vi "xml_to_dictionary.vi"(8 "error in (no error)":errorcluster, 11 "XML File Path":path) -> (0 "error out":errorcluster, 3 "units []":T1[](array[typedef]))   [LabVIEW 2015, in "lv-unit-conversion.lvlib"]
uses:
  lv-unit-conversion.lvlib
  public/_controls/unit.ctl
  public/_controls/error.ctl
  <vilib>/xml/Load XML File.vi
  <vilib>/xml/Close Reference(Node).vi
  <vilib>/xml/NI_XML.lvlib
  <resource>/objmgr/DOMUserDefRef.rc
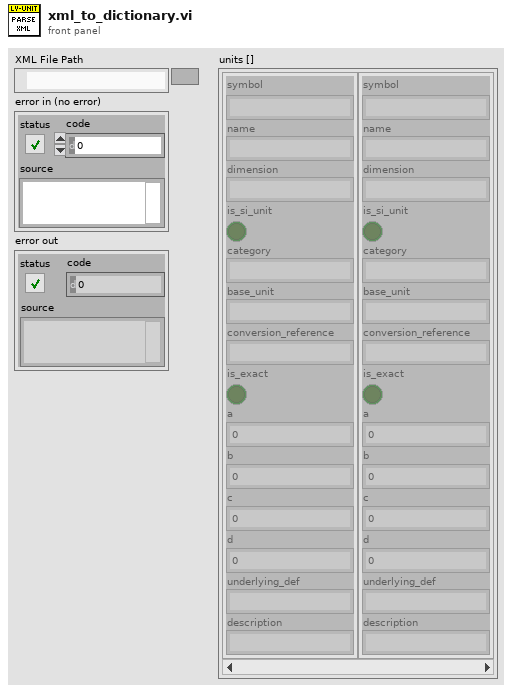
[diagram p1: front panel]
types:
  T1 = typedef "lv-unit-conversion.lvlib/unit.ctl" = cluster{"symbol":string, "name":string, "dimension":string, "is_si_unit":bool, "category":string, "base_unit":string, "conversion_reference":string, "is_exact":bool, "a":dbl, "b":dbl, "c":dbl, "d":dbl, "underlying_def":string, "description":string}
  T2 = typedef "lv-unit-conversion.lvlib/error.ctl" = enum16{"<lv-unit-conversion_error>", "unit_not_found", "xml_parser", "<null>"}
  T3 = cluster{cluster{"Name":string, "Value":string}[]}
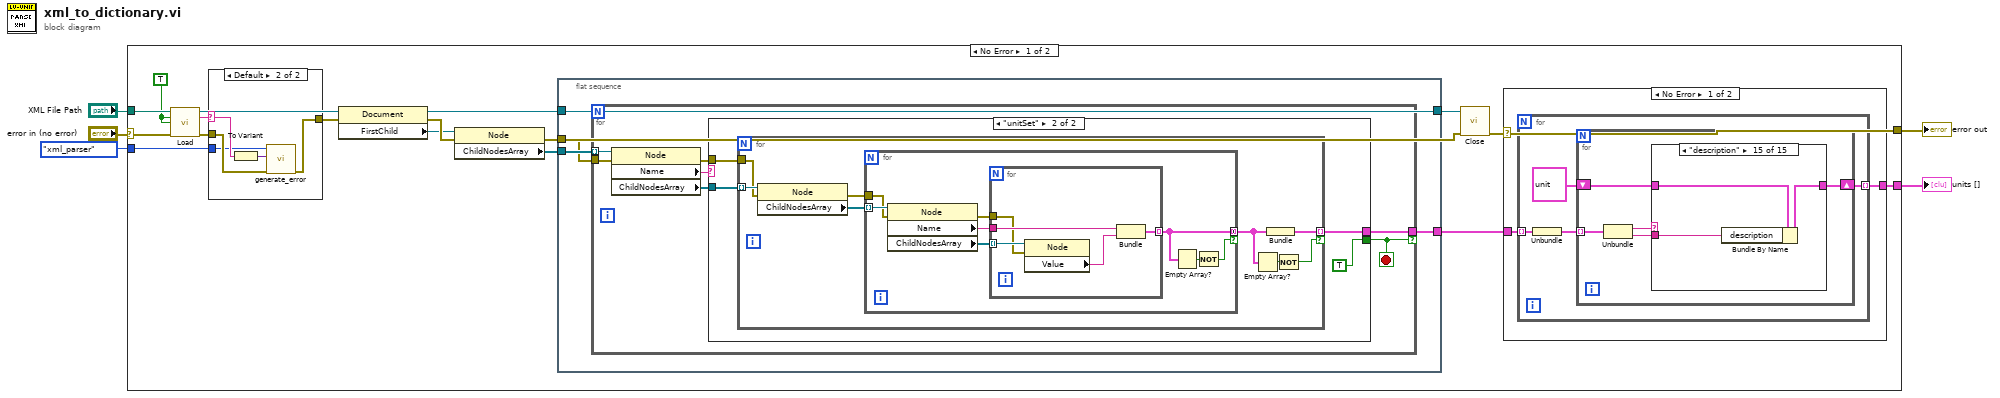
[diagram p0: block diagram]
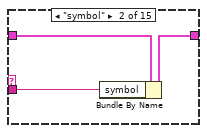
[diagram p3: hidden frame]
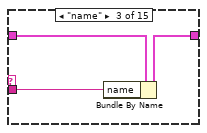
[diagram p4: hidden frame]
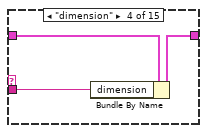
[diagram p5: hidden frame]
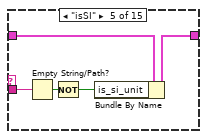
[diagram p6: hidden frame]
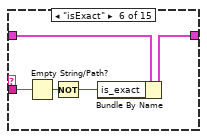
[diagram p7: hidden frame]
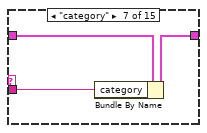
[diagram p8: hidden frame]
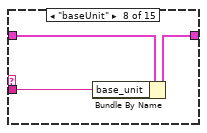
[diagram p9: hidden frame]
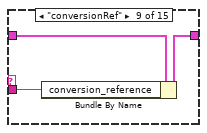
[diagram p10: hidden frame]
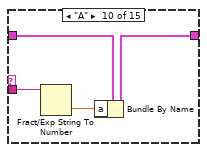
[diagram p11: hidden frame]
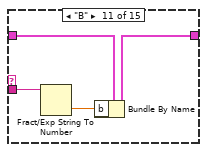
[diagram p12: hidden frame]
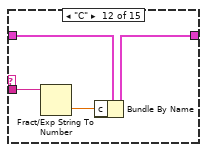
[diagram p13: hidden frame]
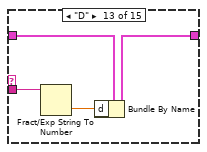
[diagram p14: hidden frame]
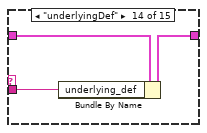
[diagram p15: hidden frame]
diagram:
  n1 = case shown="No Error" "error in (no error)" {
    selector: "error in (no error)" -> [w13 w127]
    tunnel: "XML File Path" -> [w22 _]
    tunnel: [w7 w127] -> w4
    tunnel: error."xml_parser" ("error") -> [w9 _]
    tunnel: [w6 _] -> w1
    frame No Error {
      w21 = TRUE ("process namespaces (False)")
      n2 = call-poly <vilib>:"Load.vi"("path to XML document"=w22, "process namespaces (False)"=w21, "process schema (False)"=w21, "error in (no error)"=w13) -> ("DOM document out"=w20:refnum<k20>, "parse errors"=w12:string, "error out"=w11:errorcluster)  [unwired: 9 in]
      n3 = case shown="Default" w12 {
        selector: w12 -> [_ w90]
        tunnel: w11 -> [w85 w89]
        tunnel: [w85 w88] -> w10
        tunnel: w9 -> [_ w87]
        frame "" {
        }
        frame Default {
          n4 = To Variant(anything=w90) -> (Variant=w86:variant)
          n5 = call "generate_error.vi"("error in (no error)"=w89, "data"=w86, "error"=w87) -> ("error out"=w88:errorcluster)  [unwired: 8 in]
        }
      }
      n6 = property class="Document"(reference=w20, error in=w10) -> (reference out=w16:refnum<k20>, error out=w18:errorcluster, "FirstChild"=w17:refnum<k20>)
      n7 = property class="Node"(reference=w17, error in=w18) -> (error out=w14:errorcluster, "ChildNodesArray"=w19:refnum<k20>[])  [unwired: 1 out]
      n8 = flat-sequence {
        tunnel: w19 -> [w94]
        tunnel: [w93] -> w8
        tunnel: w16 -> [w92]
        tunnel: [w92] -> w15
        tunnel: w14 -> [w91]
        frame #0 {
          n9 = for {
            tunnel: w94 -> [w101] mode=indexing
            tunnel: [w97] -> w93 if=w95
            tunnel: w91 -> [w100]
            stop <- w95 stop-if-true
            n10 = property class="Node"(reference=w101, error in=w100) -> (error out=w98:errorcluster, "Name"=w96:string, "ChildNodesArray"=w99:refnum<k20>[])  [unwired: 1 out]
            n11 = case shown="\"unitSet\"" w96 {
              tunnel: w99 -> [_ w105]
              tunnel: w98 -> [_ w104]
              tunnel: [_ w103] -> w97
              tunnel: [_ TRUE] -> w95
              frame "False", Default {
              }
              frame "unitSet" {
                n12 = for {
                  tunnel: w105 -> [w113] mode=indexing
                  tunnel: [w109] -> w103 mode=indexing if=w110
                  tunnel: w104 -> [w107]
                  n13 = property class="Node"(reference=w113, error in=w107) -> (error out=w106:errorcluster, "ChildNodesArray"=w112:refnum<k20>[])  [unwired: 1 out]
                  n14 = for {
                    tunnel: w112 -> [w121] mode=indexing
                    tunnel: [w117] -> w108 mode=concatenating if=w116
                    tunnel: w106 -> [w115]
                    n15 = property class="Node"(reference=w121, error in=w115) -> (error out=w114:errorcluster, "Name"=w119:string, "ChildNodesArray"=w120:refnum<k20>[])  [unwired: 1 out]
                    n16 = for {
                      tunnel: w120 -> [w126] mode=indexing
                      tunnel: w119 -> [w123]
                      tunnel: [w124] -> w117 mode=indexing
                      tunnel: w114 -> [w122]
                      n17 = property class="Node"(reference=w126, error in=w122) -> ("Value"=w125:string)  [unwired: 2 out]
                      n18 = Bundle("Name"=w123, "Value"=w125) -> (w124:cluster{"Name":string, "Value":string})  [unwired: 1 in]
                    }
                    n19 = Empty Array?(array=w117) -> (empty?=w118:bool)
                    n20 = Not(x=w118) -> (.not. x?=w116:bool)
                  }
                  n21 = Empty Array?(array=w108) -> (empty?=w111:bool)
                  n22 = Bundle(w108) -> (w109:T3)  [unwired: 1 in]
                  n23 = Not(x=w111) -> (.not. x?=w110:bool)
                }
              }
            }
          }
        }
      }
      n24 = call-poly <vilib>:"Close.vi"("error in (no error)"=w14, "node"=w15) -> ("error out"=w7:errorcluster)  [unwired: 7 in]
      n25 = case shown="No Error" w7 {
        tunnel: w8 -> [w23 _]
        tunnel: [w24 _] -> w6
        frame No Error {
          n26 = for {
            tunnel: w23 -> [w28] mode=indexing
            tunnel: [w25] -> w24 mode=indexing
            n27 = Unbundle(w28) -> (w27:cluster{"Name":string, "Value":string}[])
            n28 = for {
              tunnel: w27 -> [w33] mode=indexing
              shift-right: [w29] -> w25
              shift-left: T1 {"symbol"="", "name"="", "dimension"="", "is_si_unit"=FALSE, "category"="", "base_unit"="", "conversion_reference"="", "is_exact"=FALSE, "a"=0.0, "b"=0.0, "c"=0.0, "d"=0.0, "underlying_def"="", "description"=""} ("unit_set") -> [w30]
              n29 = Unbundle(w33) -> ("Name"=w32:string, "Value"=w31:string)
              n30 = case shown="\"description\"" w32 {
                tunnel: w31 -> [_ w35 w38 w41 w46 w51 w54 w57 w60 w64 w68 w72 w76 w79 w82]
                tunnel: w30 -> [w34 w37 w40 w43 w48 w53 w56 w59 w62 w66 w70 w74 w78 w81 w84]
                tunnel: [w34 w36 w39 w42 w47 w52 w55 w58 w61 w65 w69 w73 w77 w80 w83] -> w29
                frame Default {
                }
                frame "symbol" {
                  n31 = Bundle By Name(cluster=w37, "symbol"=w35) -> (w36:T1)
                }
                frame "name" {
                  n32 = Bundle By Name(cluster=w40, "name"=w38) -> (w39:T1)
                }
                frame "dimension" {
                  n33 = Bundle By Name(cluster=w43, "dimension"=w41) -> (w42:T1)
                }
                frame "isSI" {
                  n34 = Empty String/Path?(string/path=w46) -> (empty?=w45:bool)
                  n35 = Not(x=w45) -> (.not. x?=w44:bool)
                  n36 = Bundle By Name(cluster=w48, "is_si_unit"=w44) -> (w47:T1)
                }
                frame "isExact" {
                  n37 = Empty String/Path?(string/path=w51) -> (empty?=w50:bool)
                  n38 = Not(x=w50) -> (.not. x?=w49:bool)
                  n39 = Bundle By Name(cluster=w53, "is_exact"=w49) -> (w52:T1)
                }
                frame "category" {
                  n40 = Bundle By Name(cluster=w56, "category"=w54) -> (w55:T1)
                }
                frame "baseUnit" {
                  n41 = Bundle By Name(cluster=w59, "base_unit"=w57) -> (w58:T1)
                }
                frame "conversionRef" {
                  n42 = Bundle By Name(cluster=w62, "conversion_reference"=w60) -> (w61:T1)
                }
                frame "A" {
                  n43 = Fract/Exp String To Number(string=w64) -> (number=w63:dbl)  [unwired: 3 in, 1 out]
                  n44 = Bundle By Name(cluster=w66, "a"=w63) -> (w65:T1)
                }
                frame "B" {
                  n45 = Fract/Exp String To Number(string=w68) -> (number=w67:dbl)  [unwired: 3 in, 1 out]
                  n46 = Bundle By Name(cluster=w70, "b"=w67) -> (w69:T1)
                }
                frame "C" {
                  n47 = Fract/Exp String To Number(string=w72) -> (number=w71:dbl)  [unwired: 3 in, 1 out]
                  n48 = Bundle By Name(cluster=w74, "c"=w71) -> (w73:T1)
                }
                frame "D" {
                  n49 = Fract/Exp String To Number(string=w76) -> (number=w75:dbl)  [unwired: 3 in, 1 out]
                  n50 = Bundle By Name(cluster=w78, "d"=w75) -> (w77:T1)
                }
                frame "underlyingDef" {
                  n51 = Bundle By Name(cluster=w81, "underlying_def"=w79) -> (w80:T1)
                }
                frame "description" {
                  n52 = Bundle By Name(cluster=w84, "description"=w82) -> (w83:T1)
                }
              }
            }
          }
        }
        frame Error {
        }
      }
    }
    frame Error {
    }
  }
  "error out" <- w4
  "units []" <- w1
